vi "AddAll Value Change.vi"(11 "References":T1) -> (0 "error out":errorcluster)   [LabVIEW 2015, in "TDMS datalogger editor node.lvclass"]
uses:
  TDMS datalogger editor node.lvclass
  <vilib>/NI/DCAF/Tag Editor Core/Table API/Table Manager/object ref.ctl
  <vilib>/NI/DCAF/Tag Editor Core/Configuration Editor/Classes/Engine Parent/Engine Parent Editor Node.lvclass
  <vilib>/NI/DCAF/Tag Editor Core/Configuration Editor/Classes/Module editor node/module editor node.lvclass
  TDMS datalogger editor node.lvclass/TDMS datalogger editor node.ctl
  <vilib>/NI/DCAF/Tag Editor Core/Table API/Table Manager/Table Manager.lvclass
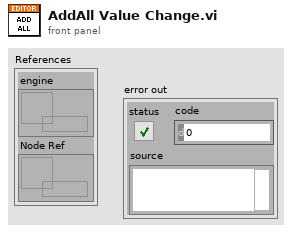
[diagram p1: front panel]
types:
  T1 = typedef "Table Manager.lvlib/Table Manager.lvclass/object ref.ctl" = cluster{"engine":refnum<data-value>, "Node Ref":refnum<data-value>}
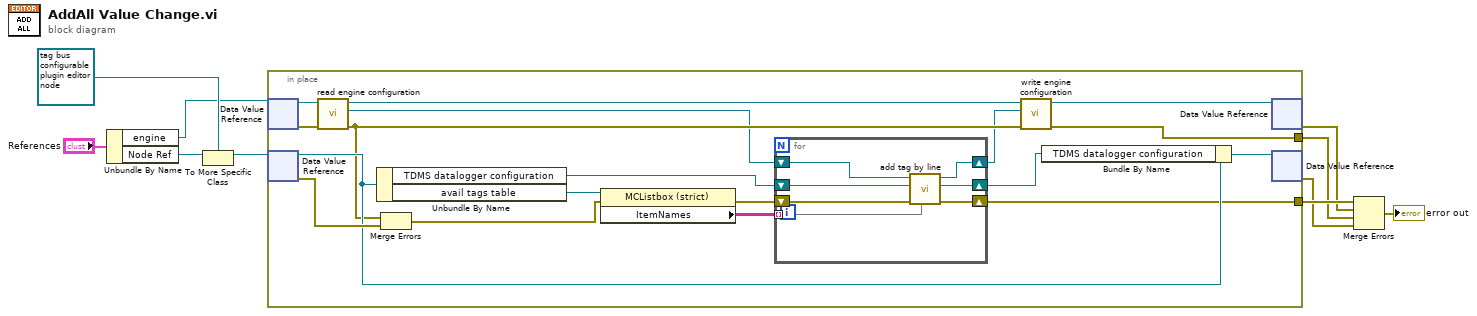
[diagram p0: block diagram]
diagram:
  n1 = Unbundle By Name("References") -> ("engine"=w2:refnum<data-value>, "Node Ref"=w5:refnum<data-value>)
  n2 = To More Specific Class(target class=refnum<data-value> refnum ("data value reference"), reference=w5) -> (specific class reference=w3:refnum<data-value>)  [unwired: 1 in, 1 out]
  n3 = in-place {
    in-place-border: [w13] -> w10
    in-place-border: [w22] -> w9
    n4 = in-place-dvr #1(w2) -> (w24:refnum<class "Engine Parent Editor Node.lvclass">, w25:errorcluster)
    n5 = in-place-dvr #2(w3) -> (w21:refnum<class "TDMS datalogger editor node.lvclass">, w27:errorcluster)
    n6 = call <vilib>:"read engine configuration.vi"("error in"=w25, "Engine Parent Editor Node in"=w24) -> ("error out"=w20:errorcluster, "engine configuration"=w15:refnum<class "engine configuration.lvclass">, "Engine Parent Editor Node out"=w23:refnum<class "Engine Parent Editor Node.lvclass">)  [unwired: 7 in]
    n7 = Unbundle By Name(w21) -> ("TDMS datalogger configuration"=w16:refnum<class "TDMS datalogger configuration.lvclass">, "avail tags table"=w11:refnum<vi>)
    n8 = Merge Errors(w20, w27) -> (w12:errorcluster)
    n9 = property on="Property Node" class="MCListbox (strict)"(reference=w11, error in=w12) -> (error out=w18:errorcluster, "ItemNames"=w19:string[][])  [unwired: 1 out]
    n10 = for {
      tunnel: w19 -> [w30] mode=indexing
      shift-right: [w34] -> w13
      shift-left: w18 -> [w32]
      shift-right: [w35] -> w17
      shift-left: w16 -> [w33]
      shift-right: [w31] -> w14
      shift-left: w15 -> [w29]
      n11 = call "add tag by line.vi"("ItemNames"=w30, "error in"=w32, "TDMS datalogger configuration in"=w33, "engine configuration in"=w29) -> ("error out"=w34:errorcluster, "TDMS datalogger configuration out"=w35:refnum<class "TDMS datalogger configuration.lvclass">, "engine configuration out"=w31:refnum<class "engine configuration.lvclass">)  [unwired: 5 in]
    }
    n12 = call <vilib>:"write engine configuration.vi"("error in"=w20, "engine configuration"=w14, "Engine Parent Editor Node in"=w23) -> ("error out"=w22:errorcluster, "Engine Parent Editor Node out"=w26:refnum<class "Engine Parent Editor Node.lvclass">)  [unwired: 7 in]
    n13 = Bundle By Name(cluster=w21, "TDMS datalogger configuration"=w17) -> (w28:refnum<class "TDMS datalogger editor node.lvclass">)
    n14 = in-place-dvr #1(w26) -> (w8:errorcluster)  [unwired: 1 out]
    n15 = in-place-dvr #2(w28) -> (w7:errorcluster)  [unwired: 1 out]
  }
  n16 = Merge Errors(w10, w8, w9, w7) -> (→"error out":errorcluster)
